vi "m s to u100m s.vi"() -> ()   [LabVIEW 2019]
panel:
  out "u/100ms":dbl
  in  "m/s":dbl
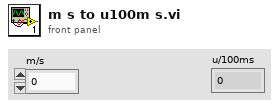
[diagram p1: front panel]
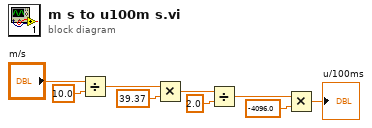
[diagram p0: block diagram]
diagram:
  n1 = Divide(x="m/s", y=10.0) -> (x/y=w8:dbl)
  n2 = Multiply(x=w8, y=39.37) -> (x*y=w5:dbl)
  n3 = Divide(x=w5, y=2.0) -> (x/y=w7:dbl)
  n4 = Multiply(x=w7, y=-4096.0) -> (x*y=→"u/100ms":dbl)
